vi "output (subVI).vi"(10 "NewVal in":bool, 11 "Boolean in":refnum<vi>) -> (2 "string out":string)   [LabVIEW 2017]
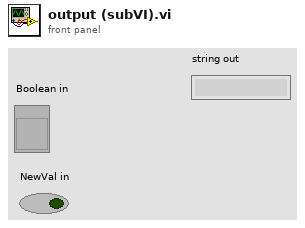
[diagram p1: front panel]
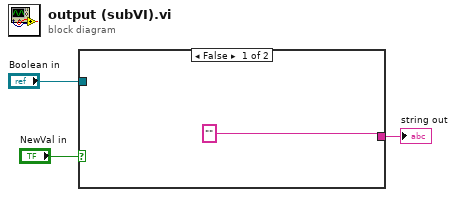
[diagram p0: block diagram]
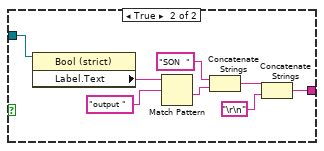
[diagram p2: hidden frame]
diagram:
  n1 = case shown="False" "NewVal in" {
    tunnel: "Boolean in" -> [_ w12]
    tunnel: ["" w5] -> w1
    frame False {
    }
    frame True {
      n2 = property class="Bool (strict)"(reference=w12) -> ("Label.Text"=w11:string)  [unwired: 1 in, 2 out]
      n3 = Match Pattern(string=w11, regular expression="output ") -> (after substring=w9:string)  [unwired: 1 in, 3 out]
      n4 = Concatenate Strings("SON  " ("String 2"), w9) -> (w7:string)
      n5 = Concatenate Strings(w7, "\r\n") -> (w5:string)
    }
  }
  "string out" <- w1
